vi "Msg.vi"(7 "jettl in":refnum<class "jettl.lvclass">, 11 "Queue Last Ack Msg Strategy in":refnum<class "Queue Last Ack Msg Strategy.lvclass">) -> (5 "jettl out":refnum<class "jettl.lvclass">)   [LabVIEW 2021, in "jettl.lvlib" / "jettl Msg Queue Last Ack.lvlib" / "Queue Last Ack Msg Strategy.lvclass"]
uses:
  Queue Last Ack Msg Strategy.lvclass
  jettl/jettl.lvclass
  Queue Last Ack/Queue Last Ack.lvclass
  Queue Last Ack Msg Strategy.lvclass/Queue Last Ack Msg Strategy.ctl
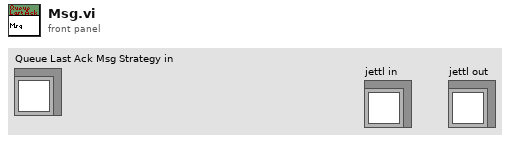
[diagram p1: front panel]
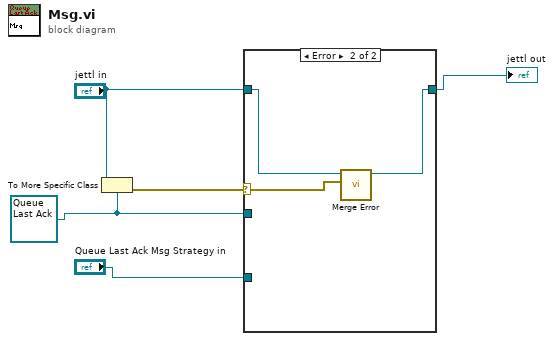
[diagram p0: block diagram]
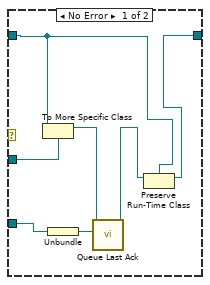
[diagram p2: hidden frame]
diagram:
  w3 = refnum<class "Queue Last Ack.lvclass"> refnum ("Last Ack.lvlib:Last Ack.lvclass")
  n1 = To More Specific Class(target class=w3, reference="jettl in") -> (error out=w5:errorcluster)  [unwired: 1 in, 1 out]
  n2 = case shown="Error" w5 {
    selector: w5 -> [_ w15]
    tunnel: [w6 w13] -> w1
    tunnel: "jettl in" -> [w8 w14]
    tunnel: w3 -> [w12 _]
    tunnel: "Queue Last Ack Msg Strategy in" -> [w10 _]
    frame No Error {
      n3 = To More Specific Class(target class=w12, reference=w8) -> (specific class reference=w11:refnum<class "Queue Last Ack.lvclass">)  [unwired: 1 in, 1 out]
      n4 = Unbundle(w10) -> (w9:refnum<class "Queue jettl.lvclass">)
      n5 = call-dynamic "Queue Last Ack.vi"("Queue jettl"=w9, "Queue Last Ack in"=w11) -> ("Queue Last Ack out"=w7:refnum<class "Queue Last Ack.lvclass">)  [unwired: 9 in]
      n6 = Preserve Run-Time Class(object in=w7, 2:w8) -> (object out=w6:refnum<class "jettl.lvclass">)  [unwired: 1 in, 1 out]
    }
    frame Error {
      n7 = call-dynamic "Merge Error.vi"("Error"=w15, "Merge Error in"=w14) -> ("Merge Error out"=w13:refnum<class "jettl.lvclass">)  [unwired: 9 in]
    }
  }
  "jettl out" <- w1
